vi "Update Axial Waveform.vi"(8 "error in (no error)":errorcluster, 11 "Model in":refnum<class "Model.lvclass">) -> (0 "error out":errorcluster, 3 "Model out":refnum<class "Model.lvclass">)   [LabVIEW 2015, in "Model.lvclass"]
uses:
  Model.lvclass
  Model.lvclass/Model.ctl
  Waveforms/Waveform/Waveform.lvclass
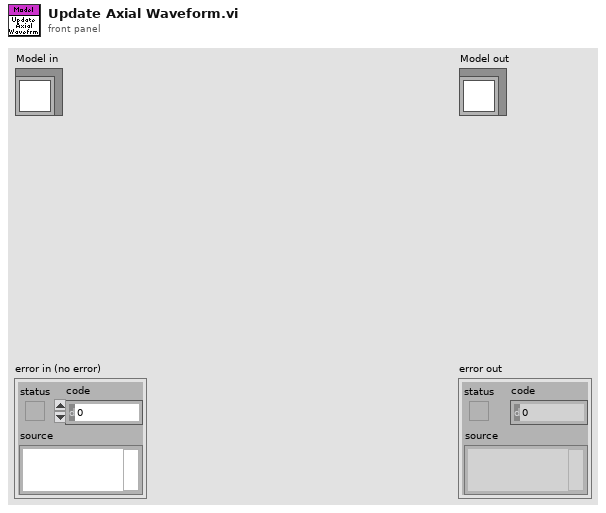
[diagram p1: front panel]
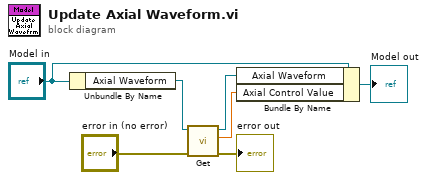
[diagram p0: block diagram]
diagram:
  n1 = Unbundle By Name("Model in") -> ("Axial Waveform"=w5:refnum<class "Waveform.lvclass">)
  n2 = call-dynamic "Get.vi"("error in (no error)"="error in (no error)", "Waveform in"=w5) -> ("error out"=→"error out":errorcluster, "Value"=w3:dbl, "Waveform out"=w4:refnum<class "Waveform.lvclass">)  [unwired: 7 in]
  n3 = Bundle By Name(cluster="Model in", "Axial Waveform"=w4, "Axial Control Value"=w3) -> (→"Model out":refnum<class "Model.lvclass">)
